vi "CNTRLR - State Process.vi"(8 "error in (no error)":errorcluster, 11 "View Model":T1) -> (0 "error out":errorcluster, 3 "View Model":T1)   [LabVIEW 2017]
doc: "This SubVI processing current CNTRLR state and decide which step will be Next"
uses:
  View Model/Controls/View Model.ctl
  View Model/Controls/Shared Model.ctl
  Error Handler/Controls/Error Model.ctl
  Error Handler/Controls/Error Message.ctl
  Error Handler/Controls/Error Level.ctl
  Configuration/Controls/Database Model.ctl
  Configuration/Controls/Database Message.ctl
  Configuration/Controls/Database Command.ctl
  Configuration/Controls/Database Overhead.ctl
  Configuration/Controls/Database Status.ctl
  Configuration/Controls/Database Record.ctl
  Configuration/Controls/Database - Rule Record.ctl
  Controls/CNTRLR - Wash Step.ctl
  Controls/CNTRLR - Position.ctl
  Controls/CNTRLR - Model.ctl
  Controls/CNTRLR - Message.ctl
  Controls/CNTRLR - Command.ctl
  Controls/CNTRLR - Overhead.ctl
  Controls/CNTRLR - State.ctl
  Controls/CNTRLR - Timer CMD.ctl
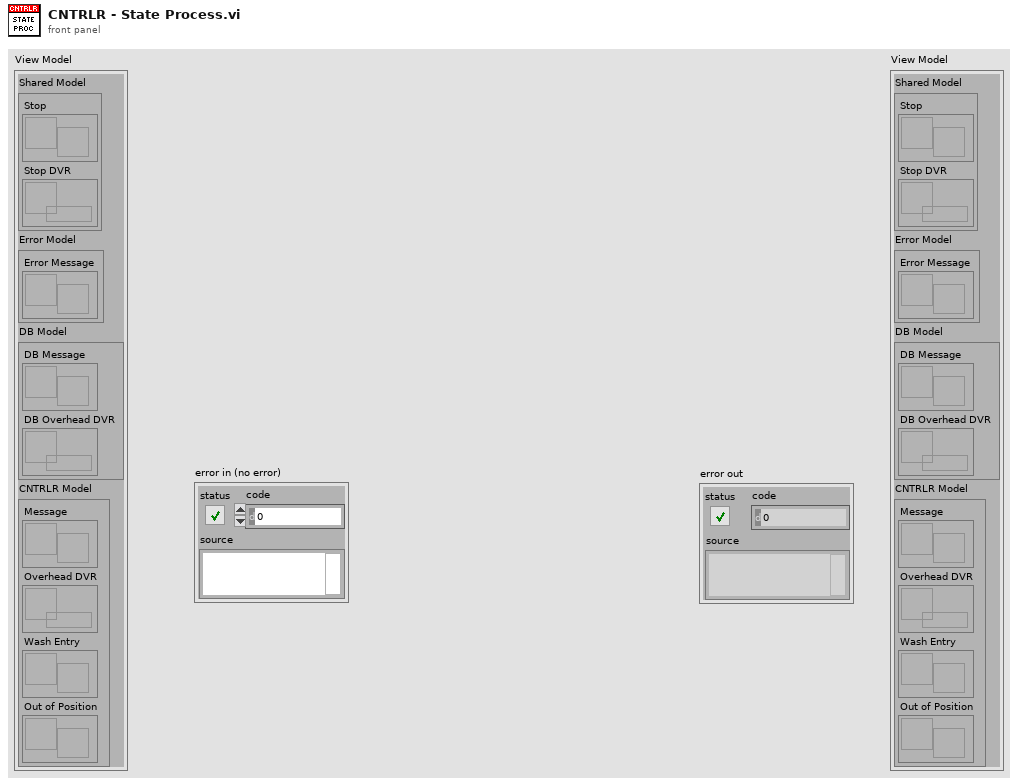
[diagram p1: front panel]
types:
  T1 = typedef "View Model.ctl" = cluster{"Shared Model":T2, "Error Model":T3, "DB Model":T4, "CNTRLR Model":T5}
  T2 = typedef "Shared Model.ctl" = cluster{"Stop":refnum<user-event>, "Stop DVR":refnum<data-value>}
  T3 = typedef "Error Model.ctl" = cluster{"Error Message":refnum<user-event>}
  T4 = typedef "Database Model.ctl" = cluster{"DB Message":refnum<user-event>, "DB Overhead DVR":refnum<data-value>}
  T5 = typedef "CNTRLR - Model.ctl" = cluster{"Message":refnum<user-event>, "Overhead DVR":refnum<data-value>, "Wash Entry":refnum<user-event>, "Out of Position":refnum<user-event>}
  T6 = typedef "Database - Rule Record.ctl" = cluster{"Wash Step":T7, "Station":T8, "Step Timing":dbl}
  T7 = typedef "CNTRLR - Wash Step.ctl" = enum16{"Under Body Wash", "Bug Remover", "Pre-Soak", "High Pressure Wash", "Low Pressure Wax", "Spot Free Rinse", "Tire Shine Foam", "Air Dry", "None"}
  T8 = typedef "CNTRLR - Position.ctl" = enum16{"Entry", "Station 1", "Station 2", "Station 3", "Exit"}
  T9 = typedef "CNTRLR - Timer CMD.ctl" = enum16{"Start", "Get Time", "Pause", "Unpause"}
  T10 = typedef "CNTRLR - State.ctl" = enum16{"Initial", "Wait for Start", "Start State", "Wait for Vehicle Position", "Wash Step Execution", "Wash Step/Cycle Complete", "Wash Exit", "Wash Abort/Terminate"}
  T11 = typedef "Database Record.ctl" = cluster{"Wash Step":string, "Station":string, "Step Duration":u32}
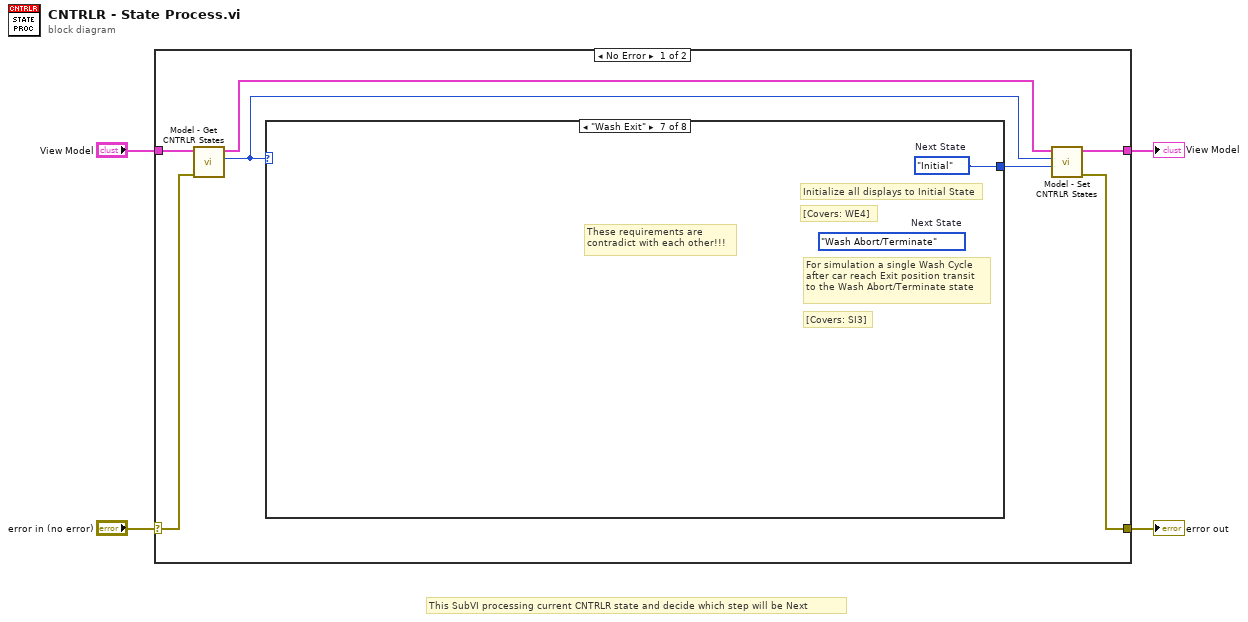
[diagram p0: block diagram]
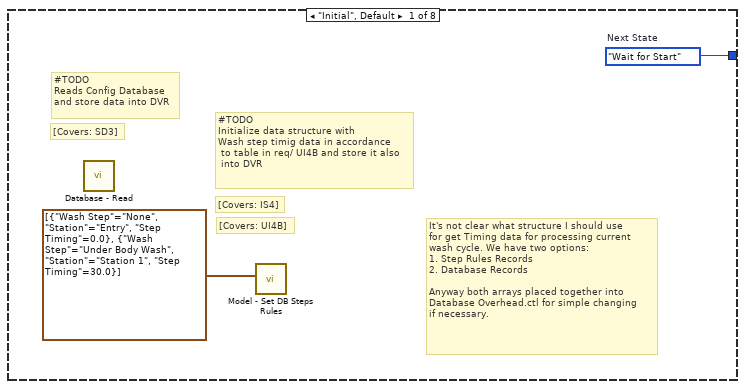
[diagram p2: hidden frame]
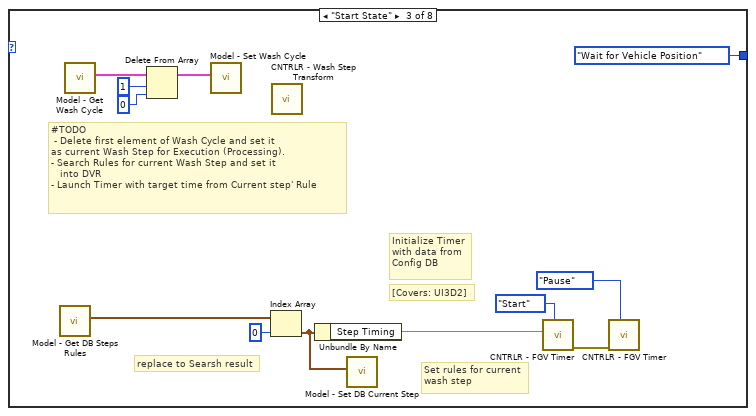
[diagram p4: hidden frame]
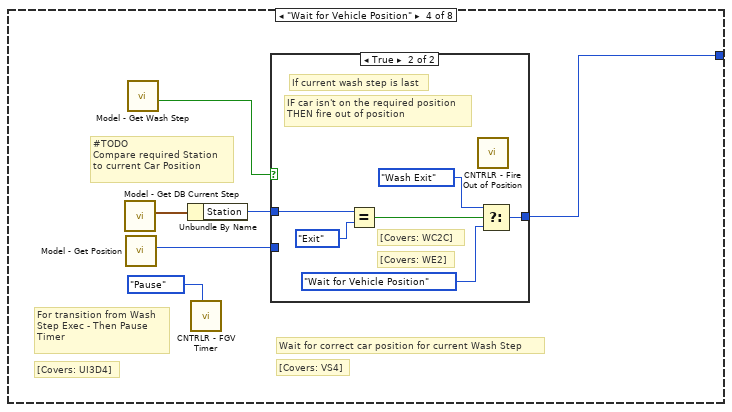
[diagram p5: hidden frame]
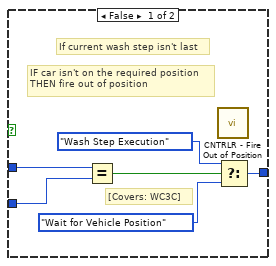
[diagram p6: hidden frame]
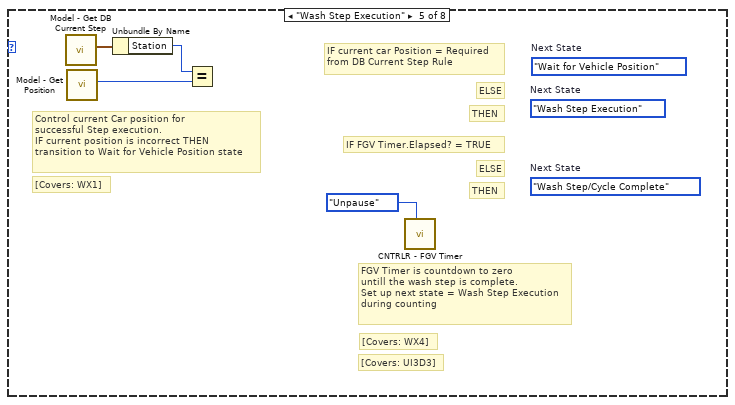
[diagram p7: hidden frame]
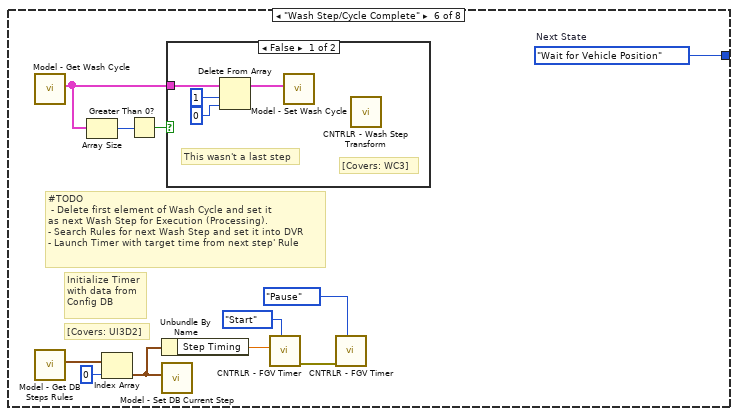
[diagram p8: hidden frame]
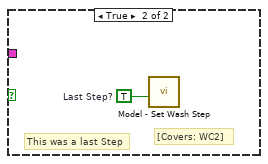
[diagram p9: hidden frame]
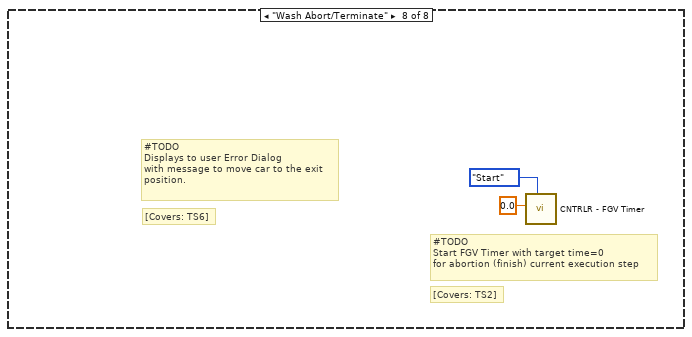
[diagram p10: hidden frame]
diagram:
  # "This SubVI processing current CNTRLR state and decide which step will be Next"
  n1 = case shown="No Error" "error in (no error)" {
    selector: "error in (no error)" -> [w11 w68]
    tunnel: [w6 w68] -> w3
    tunnel: "View Model" -> [w10 w67]
    tunnel: [w7 w67] -> w1
    frame No Error {
      n2 = call "Model - Get CNTRLR States.vi"("error in (no error)"=w11, "View Model"=w10) -> ("Current State"=w8:T10, "View Model"=w9:T1)  [unwired: 6 in, 2 out]
      n3 = case shown="\"Wash Exit\"" w8 {
        tunnel: [w12 _ CNTRLR_-_State."Wait for Vehicle Position" ("Next State") w28 _ w48 w64 _] -> w5
        frame "Initial", Default {
          w12 = CNTRLR_-_State."Wait for Start"  # Next State
          # "[Covers: UI4B]"
          # "It's not clear what structure I should use\nfor get Timing data for processing current\nwash cycle. We have two options:\n1. Step Rules Records\n2. Database Records\n\nAnyway both arrays placed together into\nDatabase Overhead.ctl for simple changing\nif necessary."
          # "[Covers: IS4]"
          # "#TODO\nInitialize data structure with\nWash step timig data in accordance\n to table in req/ UI4B and store it also\n into DVR"
          # "[Covers: SD3]"
          # "#TODO\nReads Config Database \nand store data into DVR"
          n4 = call "Database - Read.vi"() -> ()  [unwired: 10 in, 2 out]
          n5 = call "Model - Set DB Steps Rules.vi"("Steps Rules"=T6[] [{"Wash Step"=enum."None", "Station"=enum."Entry", "Step Timing"=0.0}, {"Wash Step"=enum."Under Body Wash", "Station"=enum."Station 1", "Step Timing"=30.0}]) -> ()  [unwired: 9 in, 2 out]
        }
        frame "Wait for Start" {
          # "[Covers: WS3]"
          # "[Covers: WS1]"
          # "Maintains Initial State Requirement\nand wait for user to press Start button"
        }
        frame "Start State" {
          # "[Covers: UI3D2]"
          # "Initialize Timer\nwith data from\nConfig DB"
          # "#TODO\n - Delete first element of Wash Cycle and set it\nas current Wash Step for Execution (Processing).\n- Search Rules for current Wash Step and set it \n   into DVR\n- Launch Timer with target time from Current step' Rule"
          # "Set rules for current\nwash step"
          # "replace to Searsh result"
          n6 = call "Model - Get DB Steps Rules.vi"() -> ("Steps Rules"=w21:T6[])  [unwired: 9 in, 2 out]
          n7 = call "Model - Get Wash Cycle.vi"() -> ("Wash Cycle"=w17:T11[])  [unwired: 9 in, 2 out]
          n8 = Delete From Array(array=w17, length=1, index=0) -> (array with subset deleted=w16:T11[])  [unwired: 1 out]
          n9 = call "Model - Set Wash Cycle.vi"("Wash Cycle"=w16) -> ()  [unwired: 9 in, 2 out]
          n10 = Index Array(array=w21, index=0) -> (element=w18:T6)
          n11 = call "CNTRLR - Wash Step Transform.vi"() -> ()  [unwired: 9 in, 3 out]
          n12 = Unbundle By Name(w18) -> ("Step Timing"=w19:dbl)
          n13 = call "Model - Set DB Current Step.vi"("Current Step Record"=w18) -> ()  [unwired: 9 in, 2 out]
          n14 = call "CNTRLR - FGV Timer.vi"("Timer CMD"=CNTRLR_-_Timer_CMD."Start", "Target Time"=w19) -> ("error out"=w23:errorcluster)  [unwired: 7 in, 2 out]
          n15 = call "CNTRLR - FGV Timer.vi"("Timer CMD"=CNTRLR_-_Timer_CMD."Pause", "error in (no error)"=w23) -> ()  [unwired: 7 in, 3 out]
        }
        frame "Wait for Vehicle Position" {
          # "[Covers: UI3D4]"
          # "For transition from Wash\nStep Exec - Then Pause\nTimer"
          # "[Covers: VS4]"
          # "Wait for correct car position for current Wash Step"
          # "#TODO\nCompare required Station \nto current Car Position"
          n16 = call "Model - Get DB Current Step.vi"() -> ("Current Step Record"=w27:T6)  [unwired: 9 in, 2 out]
          n17 = call "Model - Get Position.vi"() -> ("Vehicle Position"=w30:T8)  [unwired: 9 in, 2 out]
          n18 = call "Model - Get Wash Step.vi"() -> ("Last Step?"=w29:bool)  [unwired: 8 in, 3 out]
          n19 = Unbundle By Name(w27) -> ("Station"=w31:T8)
          n20 = call "CNTRLR - FGV Timer.vi"("Timer CMD"=CNTRLR_-_Timer_CMD."Pause") -> ()  [unwired: 8 in, 3 out]
          n21 = case shown="True" w29 {
            tunnel: w31 -> [w37 w43]
            tunnel: w30 -> [w36 _]
            tunnel: [w32 w39] -> w28
            frame False {
              # "[Covers: WC3C]"
              # "IF car isn't on the required position\nTHEN fire out of position"
              # "If current wash step isn't last"
              n22 = Equal?(x=w37, y=w36) -> (x = y?=w34:bool)
              n23 = call "CNTRLR - Fire Out of Position.vi"() -> ()  [unwired: 11 in, 1 out]
              n24 = Select(t=CNTRLR_-_State."Wash Step Execution" ("Next State"), s=w34, f=CNTRLR_-_State."Wait for Vehicle Position" ("Next State")) -> (s? t:f=w32:T10)
            }
            frame True {
              # "[Covers: WE2]"
              # "[Covers: WC2C]"
              # "IF car isn't on the required position\nTHEN fire out of position"
              # "If current wash step is last"
              n25 = Equal?(x=w43, y=CNTRLR_-_Position."Exit") -> (x = y?=w41:bool)
              n26 = call "CNTRLR - Fire Out of Position.vi"() -> ()  [unwired: 11 in, 1 out]
              n27 = Select(t=CNTRLR_-_State."Wash Exit" ("Next State"), s=w41, f=CNTRLR_-_State."Wait for Vehicle Position" ("Next State")) -> (s? t:f=w39:T10)
            }
          }
        }
        frame "Wash Step Execution" {
          (unwired) CNTRLR_-_State."Wash Step/Cycle Complete"  # Next State
          (unwired) CNTRLR_-_State."Wash Step Execution"  # Next State
          (unwired) CNTRLR_-_State."Wait for Vehicle Position"  # Next State
          # "[Covers: UI3D3]"
          # "ELSE"
          # "THEN"
          # "IF FGV Timer.Elapsed? = TRUE"
          # "ELSE"
          # "THEN"
          # "IF current car Position = Required\nfrom DB Current Step Rule"
          # "[Covers: WX4]"
          # "FGV Timer is countdown to zero\nuntill the wash step is complete.\nSet up next state = Wash Step Execution\nduring counting"
          # "[Covers: WX1]"
          # "Control current Car position for\nsuccessful Step execution. \nIF current position is incorrect THEN\ntransition to Wait for Vehicle Position state"
          n28 = call "Model - Get DB Current Step.vi"() -> ("Current Step Record"=w46:T6)  [unwired: 9 in, 2 out]
          n29 = call "Model - Get Position.vi"() -> ("Vehicle Position"=w44:T8)  [unwired: 9 in, 2 out]
          n30 = Unbundle By Name(w46) -> ("Station"=w45:T8)
          n31 = Equal?(x=w45, y=w44) -> ()  [unwired: 1 out]
          n32 = call "CNTRLR - FGV Timer.vi"("Timer CMD"=CNTRLR_-_Timer_CMD."Unpause") -> ()  [unwired: 8 in, 3 out]
        }
        frame "Wash Step/Cycle Complete" {
          w48 = CNTRLR_-_State."Wait for Vehicle Position"  # Next State
          # "[Covers: UI3D2]"
          # "Initialize Timer\nwith data from\nConfig DB"
          # "#TODO\n - Delete first element of Wash Cycle and set it\nas next Wash Step for Execution (Processing).\n- Search Rules for next Wash Step and set it into DVR\n- Launch Timer with target time from next step' Rule"
          n33 = call "Model - Get Wash Cycle.vi"() -> ("Wash Cycle"=w56:T11[])  [unwired: 9 in, 2 out]
          n34 = call "Model - Get DB Steps Rules.vi"() -> ("Steps Rules"=w55:T6[])  [unwired: 9 in, 2 out]
          n35 = Array Size(array=w56) -> (size(s)=w58:i32)
          n36 = Index Array(array=w55, index=0) -> (element=w54:T6)
          n37 = Greater Than 0?(x=w58) -> (x > 0?=w57:bool)
          n38 = Unbundle By Name(w54) -> ("Step Timing"=w50:dbl)
          n39 = call "Model - Set DB Current Step.vi"("Current Step Record"=w54) -> ()  [unwired: 9 in, 2 out]
          n40 = case shown="False" w57 {
            tunnel: w56 -> [w59 _]
            frame False {
              # "[Covers: WC3]"
              # "This wasn't a last step"
              n41 = Delete From Array(array=w59, length=1, index=0) -> (array with subset deleted=w62:T11[])  [unwired: 1 out]
              n42 = call "Model - Set Wash Cycle.vi"("Wash Cycle"=w62) -> ()  [unwired: 9 in, 2 out]
              n43 = call "CNTRLR - Wash Step Transform.vi"() -> ()  [unwired: 9 in, 3 out]
            }
            frame True {
              w63 = TRUE  # Last Step?
              # "[Covers: WC2]"
              # "This was a last Step"
              n44 = call "Model - Set Wash Step.vi"("Last Step?"=w63) -> ()  [unwired: 9 in, 2 out]
            }
          }
          n45 = call "CNTRLR - FGV Timer.vi"("Timer CMD"=CNTRLR_-_Timer_CMD."Start", "Target Time"=w50) -> ("error out"=w49:errorcluster)  [unwired: 7 in, 2 out]
          n46 = call "CNTRLR - FGV Timer.vi"("Timer CMD"=CNTRLR_-_Timer_CMD."Pause", "error in (no error)"=w49) -> ()  [unwired: 7 in, 3 out]
        }
        frame "Wash Exit" {
          (unwired) CNTRLR_-_State."Wash Abort/Terminate"  # Next State
          w64 = CNTRLR_-_State."Initial"  # Next State
          # "These requirements are\ncontradict with each other!!!"
          # "[Covers: SI3]"
          # "For simulation a single Wash Cycle\nafter car reach Exit position transit\nto the Wash Abort/Terminate state"
          # "[Covers: WE4]"
          # "Initialize all displays to Initial State"
        }
        frame "Wash Abort/Terminate" {
          # "[Covers: TS2]"
          # "#TODO\nStart FGV Timer with target time=0\nfor abortion (finish) current execution step"
          # "[Covers: TS6]"
          # "#TODO\nDisplays to user Error Dialog\nwith message to move car to the exit\nposition."
          n47 = call "CNTRLR - FGV Timer.vi"("Timer CMD"=CNTRLR_-_Timer_CMD."Start", "Target Time"=0.0) -> ()  [unwired: 7 in, 3 out]
        }
      }
      n48 = call "Model - Set CNTRLR States.vi"("Next State"=w5, "Current State"=w8, "View Model"=w9) -> ("error out"=w6:errorcluster, "View Model"=w7:T1)  [unwired: 7 in]
    }
    frame Error {
    }
  }
  "error out" <- w3
  "View Model" <- w1
